vi "Initialize Aliases Page.vi"(8 "error in (no error)":errorcluster, 10 "Aliases Page Controls":T1, 11 "Aliases Ref in":T2 format="%.0x") -> (0 "error out":errorcluster, 3 "Aliases Ref out":T2 format="%.0x")   [LabVIEW 2017, in "Routing and Faulting System Explorer.lvlib"]
uses:
  Routing and Faulting System Explorer.lvlib
  <vilib>/NI Veristand/Custom Device API/Custom Device Item Ref.ctl
  Aliases Page Controls.ctl
  Alias.ctl
  Endpoint.ctl
  Scripting/Routing and Faulting Scripting.lvlib
  <vilib>/NI Veristand/Custom Device API/Custom Device API.lvlib
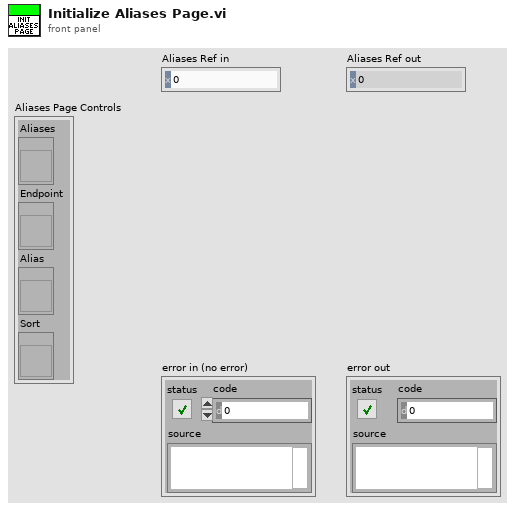
[diagram p1: front panel]
types:
  T1 = typedef "Routing and Faulting System Explorer.lvlib/Aliases Page Controls.ctl" = cluster{"Aliases":refnum<vi>, "Endpoint":refnum<vi>, "Alias":refnum<vi>, "Sort":refnum<vi>}
  T2 = typedef "Custom Device API.lvlib/Custom Device Item Ref.ctl" = u64
  T3 = enum8{"Enabled", "Disabled", "Disabled and Grayed Out"}
  T4 = typedef "Routing and Faulting Shared.lvlib/Alias Mapping.ctl" = cluster{"Endpoint":string, "Alias":string}
  T5 = typedef "Routing and Faulting System Explorer.lvlib/Alias.ctl" = cluster{"Endpoint":T6, "Alias":string, "Remove":bool}
  T6 = typedef "Routing and Faulting System Explorer.lvlib/Endpoint.ctl" = string
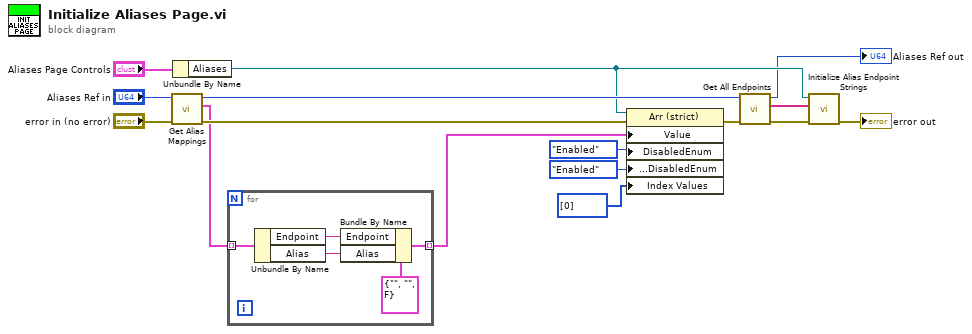
[diagram p0: block diagram]
diagram:
  n1 = call "Get Alias Mappings.vi"("error in (no error)"="error in (no error)", "Endpoint Aliases Ref in"="Aliases Ref in") -> ("error out"=w11:errorcluster, "Alias Mappings"=w10:T4[], "Endpoint Aliases Ref out"=w7:T2)  [unwired: 7 in]
  n2 = Unbundle By Name("Aliases Page Controls") -> ("Aliases"=w3:refnum<vi>)
  n3 = for {
    tunnel: w10 -> [w18] mode=indexing
    tunnel: [w17] -> w8 mode=indexing
    n4 = Unbundle By Name(w18) -> ("Endpoint"=w20:string, "Alias"=w21:string)
    n5 = Bundle By Name(cluster=T5 {"Endpoint"="", "Alias"="", "Remove"=FALSE} ("Alias"), "Endpoint"=w20, "Alias"=w21) -> (w17:T5)
  }
  n6 = property class="Arr (strict)"(reference=w3, error in=w11, "Value"=w8, "DisabledEnum"=T3."Enabled" ("Disabled"), "Array Element.DisabledEnum"=T3."Enabled" ("Array Element.Disabled"), "Index Values"=u32[] [0]) -> (error out=w6:errorcluster)  [unwired: 1 out]
  n7 = call "Get All Endpoints.vi"("error in (no error)"=w6, "Aliases Ref in"=w7) -> ("error out"=w5:errorcluster, "Addressable Endpoints"=w4:string[], "Aliases Ref out"=→"Aliases Ref out":T2)  [unwired: 7 in]
  n8 = call "Initialize Alias Endpoint Strings.vi"("error in (no error)"=w5, "Endpoints"=w4, "Aliases Ctl Ref"=w3) -> ("error out"=→"error out":errorcluster)  [unwired: 7 in, 1 out]
